vi "Execute Logging Command.vi"(8 "error in (no error)":errorcluster, 10 "command":T1={"Command"=enum."Log Plugin State", "Parameters"={"arg1"=0, "arg2"=0}}, 11 "Logging Thread in":refnum<class "Logging Thread.lvclass">) -> (0 "error out":errorcluster, 3 "Logging Thread out":refnum<class "Logging Thread.lvclass">)   [LabVIEW 2017, in "DSF Core.lvlib" / "Logging Thread.lvclass"]
uses:
  Logging Thread.lvclass
  C:/Git/DSF/Core/Classes/Thread/Thread.lvclass
  Interface/Logging/Command Data.ctl
  Interface/Logging/Command.ctl
  Interface/Logging/Parameters.ctl
  Logging Thread.lvclass/Logging Thread.ctl
  Interface/Logging/Response Data.ctl
  Interface/Logging/Response.ctl
  Interface/Logging/Framework State Parameters.ctl
  Framework/Framework States.ctl
  Pointers/Error/Error Pointer.lvclass
  C:/Program Files (x86)/National Instruments/LabVIEW 2017/vi.lib/NI/Memory Manager/Classes/Pointer/Pointer.lvclass
  <vilib>/NI/Memory Manager/Classes/Pointer/Pointer.lvclass/Pointer.ctl
  Interface/Logging/Plugin State Parameters.ctl
  Interface/Plugin/Command.ctl
  Interface/Logging/Dispatcher State Parameters.ctl
  Interface/Dispatcher/Command.ctl
  <vilib>/NI/Memory Manager/Classes/Pointer/Set Size.vi
  <vilib>/NI/Memory Manager/Classes/Pointer/Set Address.vi
  <vilib>/NI/Memory Manager/Classes/Pointer/Check Null Pointer.vi
  <vilib>/NI/Memory Manager/Classes/Pointer/Set Internal.vi
  <vilib>/NI/Memory Manager/Classes/Pointer/Errors.vi
  <vilib>/NI/Memory Manager/Classes/Pointer/Null Pointer.vi
  <vilib>/NI/Memory Manager/Classes/Pointer/Is Null.vi
  <vilib>/NI/Memory Manager/Classes/Pointer/Create Error.vi
  <vilib>/NI/Memory Manager/Classes/Pointer/Get Address.vi
  <vilib>/NI/Memory Manager/Constants/Constants.vi
  <vilib>/NI/Memory Manager/Constants/Library Name.vi
  <vilib>/NI/Memory Manager/Classes/Pointer/Pointer Error Info.vi
  <vilib>/NI/Memory Manager/Constants/Pointer Class Name.vi
  Interface/Logging/Send Logging Response.vi
  <vilib>/NI/Memory Manager/VIs/New Error Cluster.vi
  <vilib>/NI/Memory Manager/VIs/New Error Cluster (512B).vi
  <vilib>/NI/Memory Manager/VIs/Set Error Status.vi
  <vilib>/NI/Memory Manager/VIs/Set Error Code.vi
  <vilib>/NI/Memory Manager/VIs/Set Error Source.vi
  <vilib>/NI/Memory Manager/VIs/Write String to Source.vi
  Thread.lvclass
  Interface/Logging/Logging Interface.lvclass
  Framework/Framework.lvclass
  Interface/Plugin/Plugin Interface.lvclass
  <vilib>/NI/Memory Manager/Classes/Pointer/Pointer.lvclass
  Interface/Dispatcher/Dispatcher Interface.lvclass
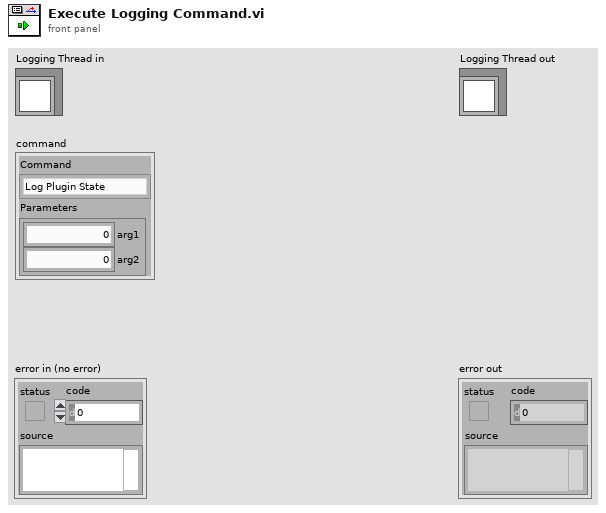
[diagram p1: front panel]
types:
  T1 = typedef "DSF Core.lvlib/Logging Interface.lvclass/Command Data.ctl" = cluster{"Command":T2, "Parameters":T3}
  T2 = typedef "DSF Core.lvlib/Logging Interface.lvclass/Command.ctl" = enum8{"Idle", "Start", "Log Framework State", "Log Plugin State", "Log Dispatcher State", "Shutdown"}
  T3 = typedef "DSF Core.lvlib/Logging Interface.lvclass/Parameters.ctl" = cluster{"arg1":u64, "arg2":u64}
  T4 = typedef "DSF Core.lvlib/Logging Interface.lvclass/Response Data.ctl" = cluster{"Response":T5, "Parameters":T3}
  T5 = typedef "DSF Core.lvlib/Logging Interface.lvclass/Response.ctl" = enum8{"General Ack", "Error", "Shutting Down"}
  T6 = typedef "DSF Core.lvlib/Logging Interface.lvclass/Framework State Parameters.ctl" = cluster{"state":T7, "unused":u8, "unused 2":u16, "unused 3":u32, "error pointer":u64}
  T7 = typedef "DSF Core.lvlib/Framework.lvclass/Framework States.ctl" = enum8{"Uninitialized", "Initialized", "Start", "Rx", "Tx", "Shutdown"}
  T8 = typedef "DSF Core.lvlib/Logging Interface.lvclass/Plugin State Parameters.ctl" = cluster{"state":T9, "Plugin ID":u8, "Thread ID":u8, "unused 0":u8, "unused 1":i32, "error pointer":u64}
  T9 = typedef "DSF Core.lvlib/Plugin Interface.lvclass/Command.ctl" = enum8{"Idle", "Start", "Set Inline Buffer", "Rx", "Tx", "Shutdown", "Error"}
  T10 = typedef "DSF Core.lvlib/Logging Interface.lvclass/Dispatcher State Parameters.ctl" = cluster{"state":T11, "unused":u8, "unused 2":u16, "unused 3":u32, "error pointer":u64}
  T11 = typedef "DSF Core.lvlib/Dispatcher Interface.lvclass/Command.ctl" = enum8{"Idle", "Start", "Rx", "Tx", "Set Inline Buffer", "Shutdown", "Error"}
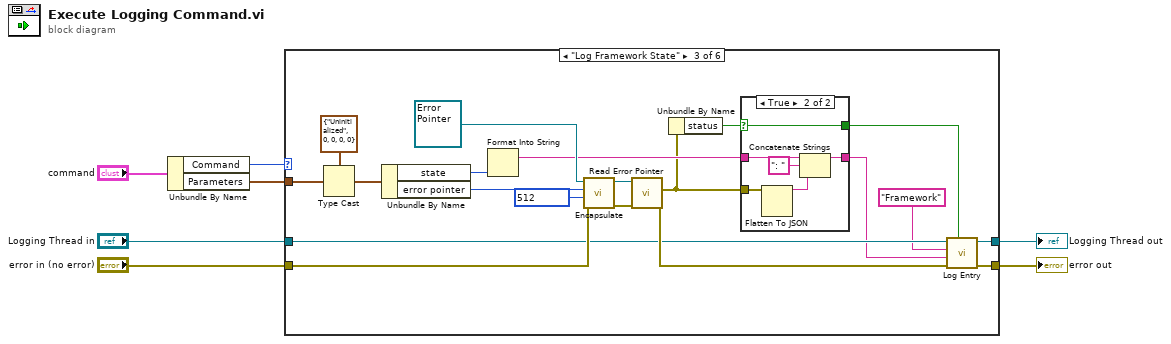
[diagram p0: block diagram]
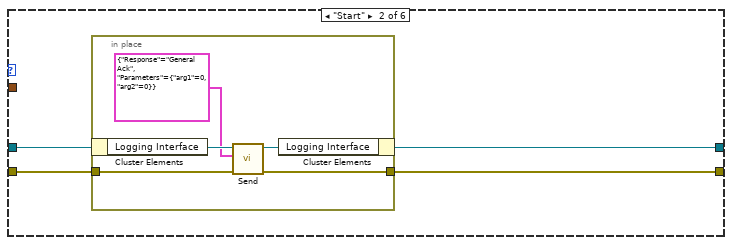
[diagram p3: hidden frame]
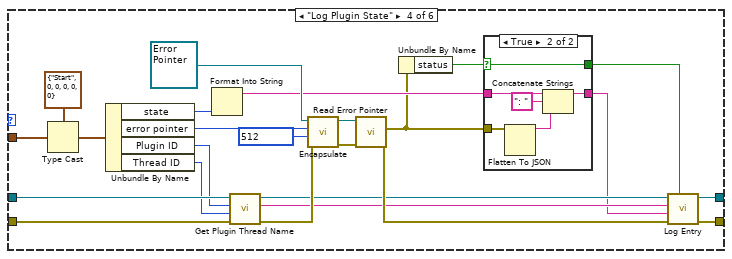
[diagram p5: hidden frame]
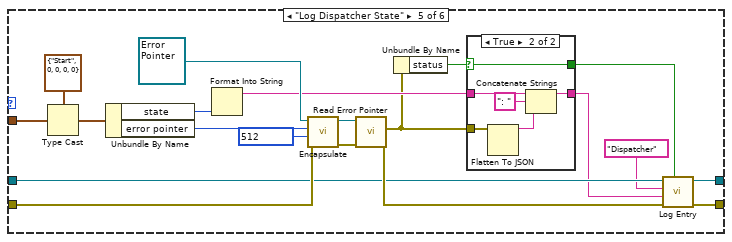
[diagram p7: hidden frame]
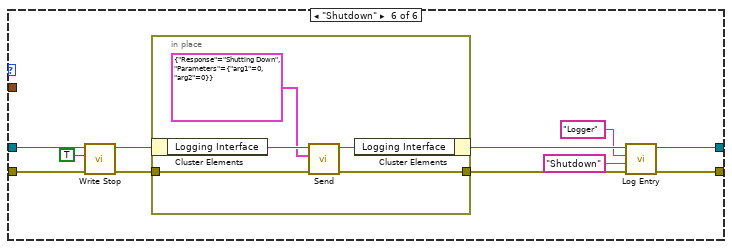
[diagram p9: hidden frame]
diagram:
  n1 = Unbundle By Name("command") -> ("Command"=w6:T2, "Parameters"=w5:T3)
  n2 = case shown="\"Log Framework State\"" w6 {
    tunnel: w5 -> [_ _ w38 w70 w98 _]
    tunnel: "Logging Thread in" -> [w9 w13 w25 w58 w85 w116]
    tunnel: [w9 w10 w33 w65 w93 w109] -> w4
    tunnel: "error in (no error)" -> [w8 w12 w32 w57 w92 w117]
    tunnel: [w8 w11 w34 w66 w94 w110] -> w3
    frame "Idle" {
    }
    frame "Start" {
      n3 = in-place {
        in-place-border: w12 -> [w16]
        in-place-border: [w15] -> w11
        n4 = in-place-cluster #1(w13) -> ("Logging Interface"=w18:refnum<class "Logging Interface.lvclass">)
        n5 = call-poly "Send.vi"("error in (no error)"=w16, "response"=T4 {"Response"=enum."General Ack", "Parameters"={"arg1"=0, "arg2"=0}}, "Logging Interface in"=w18) -> ("error out"=w15:errorcluster, "Logging Interface out"=w17:refnum<class "Logging Interface.lvclass">)  [unwired: 7 in]
        n6 = in-place-cluster #1("Logging Interface"=w17) -> (w10:refnum<class "Logging Thread.lvclass">)
      }
    }
    frame "Log Framework State" {
      n7 = Type Cast(type=T6 {"state"=enum."Uninitialized", "unused"=0, "unused 2"=0, "unused 3"=0, "error pointer"=0} ("Parameters"), x=w38) -> (*(type *) &x=w36:T6)
      n8 = Unbundle By Name(w36) -> ("state"=w35:T7, "error pointer"=w31:u64)
      n9 = Format Into String(w35) -> (resulting string=w24:string)  [unwired: 3 in, 1 out]
      n10 = call <vilib>:"Encapsulate.vi"("error in (no error)"=w32, "size"=u64 512, "address"=w31, "Pointer type"=refnum<class "Error Pointer.lvclass"> refnum ("DSF Core.lvlib:Error Pointer.lvclass")) -> ("error out"=w27:errorcluster, "Pointer"=w28:refnum<class "Error Pointer.lvclass">)  [unwired: 6 in]
      n11 = call "Read Error Pointer.vi"("error in (no error)"=w27, "Error Pointer in"=w28) -> ("error out"=w26:errorcluster, "error"=w21:errorcluster)  [unwired: 7 in, 1 out]
      n12 = Unbundle By Name(w21) -> ("status"=w20:bool)
      n13 = case shown="True" w20 {
        selector: w20 -> [w39 w42]
        tunnel: w24 -> [w40 w41]
        tunnel: [w40 w44] -> w23
        tunnel: w21 -> [_ w43]
        tunnel: [w39 w42] -> w19
        frame False {
        }
        frame True {
          n14 = Flatten To JSON(anything=w43) -> (JSON string=w45:string)  [unwired: 2 in, 1 out]
          n15 = Concatenate Strings(w41, ": " ("string"), w45) -> (w44:string)
        }
      }
      n16 = call "Log Entry.vi"("error? (F)"=w19, "error in (no error)"=w26, "line text"=w23, "line tag"="Framework", "Logging Thread in"=w25) -> ("error out"=w34:errorcluster, "Logging Thread out"=w33:refnum<class "Logging Thread.lvclass">)  [unwired: 5 in]
    }
    frame "Log Plugin State" {
      n17 = Type Cast(type=T8 {"state"=enum."Start", "Plugin ID"=0, "Thread ID"=0, "unused 0"=0, "unused 1"=0, "error pointer"=0} ("Parameters"), x=w70) -> (*(type *) &x=w68:T8)
      n18 = Unbundle By Name(w68) -> ("state"=w67:T9, "error pointer"=w64:u64, "Plugin ID"=w54:u8, "Thread ID"=w55:u8)
      n19 = Format Into String(w67) -> (resulting string=w51:string)  [unwired: 3 in, 1 out]
      n20 = call "Get Plugin Thread Name.vi"("error in (no error)"=w57, "Thread ID"=w55, "Plugin ID"=w54, "Logging Thread in"=w58) -> ("error out"=w56:errorcluster, "thread name"=w52:string, "Logging Thread out"=w53:refnum<class "Logging Thread.lvclass">)  [unwired: 5 in]
      n21 = call <vilib>:"Encapsulate.vi"("error in (no error)"=w56, "size"=u64 512, "address"=w64, "Pointer type"=refnum<class "Error Pointer.lvclass"> refnum ("DSF Core.lvlib:Error Pointer.lvclass")) -> ("error out"=w60:errorcluster, "Pointer"=w61:refnum<class "Error Pointer.lvclass">)  [unwired: 6 in]
      n22 = call "Read Error Pointer.vi"("error in (no error)"=w60, "Error Pointer in"=w61) -> ("error out"=w59:errorcluster, "error"=w48:errorcluster)  [unwired: 7 in, 1 out]
      n23 = Unbundle By Name(w48) -> ("status"=w50:bool)
      n24 = case shown="True" w50 {
        selector: w50 -> [w71 w74]
        tunnel: w51 -> [w72 w73]
        tunnel: [w72 w76] -> w47
        tunnel: w48 -> [_ w75]
        tunnel: [w71 w74] -> w49
        frame False {
        }
        frame True {
          n25 = Flatten To JSON(anything=w75) -> (JSON string=w77:string)  [unwired: 2 in, 1 out]
          n26 = Concatenate Strings(w73, ": " ("string"), w77) -> (w76:string)
        }
      }
      n27 = call "Log Entry.vi"("error? (F)"=w49, "error in (no error)"=w59, "line text"=w47, "line tag"=w52, "Logging Thread in"=w53) -> ("error out"=w66:errorcluster, "Logging Thread out"=w65:refnum<class "Logging Thread.lvclass">)  [unwired: 5 in]
    }
    frame "Log Dispatcher State" {
      n28 = Type Cast(type=T10 {"state"=enum."Start", "unused"=0, "unused 2"=0, "unused 3"=0, "error pointer"=0} ("Parameters"), x=w98) -> (*(type *) &x=w96:T10)
      n29 = Unbundle By Name(w96) -> ("state"=w95:T11, "error pointer"=w91:u64)
      n30 = Format Into String(w95) -> (resulting string=w83:string)  [unwired: 3 in, 1 out]
      n31 = call <vilib>:"Encapsulate.vi"("error in (no error)"=w92, "size"=u64 512, "address"=w91, "Pointer type"=refnum<class "Error Pointer.lvclass"> refnum ("DSF Core.lvlib:Error Pointer.lvclass")) -> ("error out"=w87:errorcluster, "Pointer"=w88:refnum<class "Error Pointer.lvclass">)  [unwired: 6 in]
      n32 = call "Read Error Pointer.vi"("error in (no error)"=w87, "Error Pointer in"=w88) -> ("error out"=w86:errorcluster, "error"=w81:errorcluster)  [unwired: 7 in, 1 out]
      n33 = Unbundle By Name(w81) -> ("status"=w82:bool)
      n34 = case shown="True" w82 {
        selector: w82 -> [w99 w102]
        tunnel: w83 -> [w100 w101]
        tunnel: [w100 w104] -> w80
        tunnel: w81 -> [_ w103]
        tunnel: [w99 w102] -> w79
        frame False {
        }
        frame True {
          n35 = Flatten To JSON(anything=w103) -> (JSON string=w105:string)  [unwired: 2 in, 1 out]
          n36 = Concatenate Strings(w101, ": " ("string"), w105) -> (w104:string)
        }
      }
      n37 = call "Log Entry.vi"("error? (F)"=w79, "error in (no error)"=w86, "line text"=w80, "line tag"="Dispatcher", "Logging Thread in"=w85) -> ("error out"=w94:errorcluster, "Logging Thread out"=w93:refnum<class "Logging Thread.lvclass">)  [unwired: 5 in]
    }
    frame "Shutdown" {
      n38 = call "Write Stop.vi"("error in (no error)"=w117, "stop"=TRUE, "Thread in"=w116) -> ("error out"=w114:errorcluster, "Thread out"=w113:refnum<class "Logging Thread.lvclass">)  [unwired: 7 in]
      n39 = in-place {
        in-place-border: w114 -> [w120]
        in-place-border: [w119] -> w111
        n40 = in-place-cluster #2(w113) -> ("Logging Interface"=w122:refnum<class "Logging Interface.lvclass">)
        n41 = call-poly "Send.vi"("error in (no error)"=w120, "response"=T4 {"Response"=enum."Shutting Down", "Parameters"={"arg1"=0, "arg2"=0}}, "Logging Interface in"=w122) -> ("error out"=w119:errorcluster, "Logging Interface out"=w121:refnum<class "Logging Interface.lvclass">)  [unwired: 7 in]
        n42 = in-place-cluster #2("Logging Interface"=w121) -> (w108:refnum<class "Logging Thread.lvclass">)
      }
      n43 = call "Log Entry.vi"("error in (no error)"=w111, "line text"="Shutdown", "line tag"="Logger", "Logging Thread in"=w108) -> ("error out"=w110:errorcluster, "Logging Thread out"=w109:refnum<class "Logging Thread.lvclass">)  [unwired: 6 in]
    }
  }
  "error out" <- w3
  "Logging Thread out" <- w4
